vi "sub_pf_localization.vi"(11 "p-val out":T2) -> ()   [LabVIEW 2019]
uses:
  <vilib>/Analysis/Matrix/Datatypes/RealMatrix.ctl
  Ctrl/cmd_common.ctl
  <vilib>/Analysis/baseanly.llb/Real A x B.vi
  <vilib>/ptbypt/NI_PtbyPt.lvlib
  <vilib>/Analysis/NI_AALBase.lvlib
  <vilib>/Analysis/Matrix/NI_Matrix.lvlib
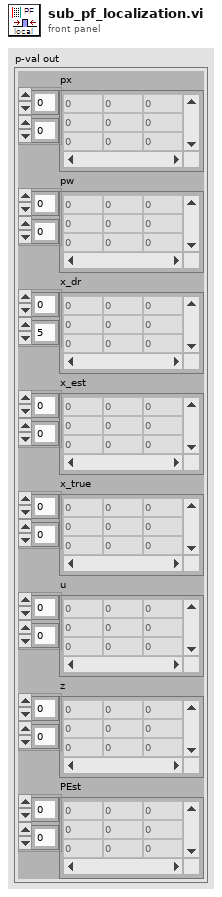
[diagram p1: front panel]
types:
  T1 = typedef "NI_Matrix.lvlib/RealMatrix.ctl" = dbl[][]
  T2 = cluster{"px":T1, "pw":T1, "x_dr":T1, "x_est":T1, "x_true":T1, "u":T1, "z":T1, "PEst":T1}
  T3 = typedef "cmd_common.ctl" = enum16{"read", "write"}
  T4 = cluster{"DT":dbl, "SIM_TIME":dbl, "MAX_RANGE":dbl, "NP":u32, "NTh":u32, "Q":T1, "R":T1, "Q_sim":T1, "R_sim":T1, "rf_id":cluster{"x":dbl, "y":dbl}[]}
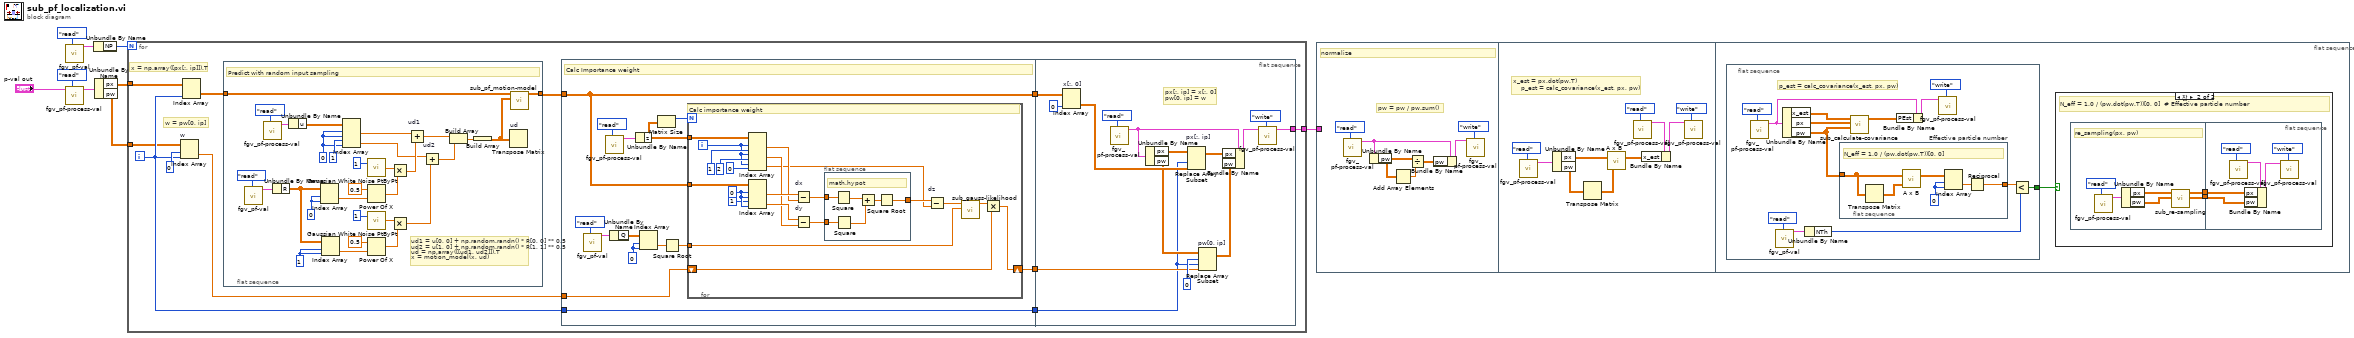
[diagram p0: block diagram]
diagram:
  n1 = call "fgv_pf-val.vi"("cmd"=cmd_common."read") -> ("pf-val out"=w7:T4)  [unwired: 10 in]
  n2 = call "fgv_pf-process-val.vi"("cmd"=cmd_common."read", "p-val"="p-val out") -> ("p-val out"=w2:T2)  [unwired: 9 in]
  n3 = Unbundle By Name(w7) -> ("NP"=w5:u32)
  n4 = Unbundle By Name(w2) -> ("px"=w4:T1, "pw"=w3:T1)
  n5 = for {
    N: w5 -> [_]
    tunnel: [w14] -> w8
    tunnel: w4 -> [w12]
    tunnel: w3 -> [w11]
    i -> [w13]
    # "x = np.array([px[:, ip]]).T"
    # "w = pw[0, ip]"
    n6 = Index Array "w"(array=w11, index (row)=0 ("인덱스 (행)"), index (col)=w13) -> (element=w18:dbl)
    n7 = Index Array(array=w12, index (col)=w13) -> (element=w10:T1)  [unwired: 1 in]
    n8 = flat-sequence {
      tunnel: [w23] -> w19
      tunnel: w10 -> [w22]
      frame #0 {
        w31 = 1 ("인덱스 (행)")
        w42 = 0 ("인덱스 (행)")
        w46 = 0 ("인덱스 (행)")
        # "ud1 = u[0, 0] + np.random.randn() * R[0, 0] ** 0.5\nud2 = u[1, 0] + np.random.randn() * R[1, 1] ** 0.5\nud = np.array([[ud1, ud2]]).T\nx = motion_model(x, ud)"
        # "Predict with random input sampling"
        n9 = call "fgv_pf-val.vi"("cmd"=cmd_common."read") -> ("pf-val out"=w43:T4)  [unwired: 10 in]
        n10 = call "fgv_pf-process-val.vi"("cmd"=cmd_common."read") -> ("p-val out"=w49:T2)  [unwired: 10 in]
        n11 = Unbundle By Name(w43) -> ("R"=w24:T1)
        n12 = Unbundle By Name(w49) -> ("u"=w48:T1)
        n13 = Index Array(array=w24, index (row)=w42, index (col)=w42) -> (element=w41:dbl)
        n14 = Index Array(array=w24, index (row)=w31, index (col)=w31) -> (element=w32:dbl)
        n15 = Index Array(array=w48, index (row) #1=w46, index (col) #1=w46, index (row) #2=1 ("인덱스 (행)"), index (col) #2=w46) -> (element #1=w36:dbl, element #2=w29:dbl)
        n16 = call <vilib>:"Gaussian White Noise PtByPt.vi"("standard deviation"=1 ("samples")) -> ("Gaussian white noise"=w38:dbl)  [unwired: 2 in]
        n17 = Power Of X(1:w41, 2:0.5 ("y")) -> (0:w39:dbl)
        n18 = call <vilib>:"Gaussian White Noise PtByPt.vi"("standard deviation"=1 ("samples")) -> ("Gaussian white noise"=w35:dbl)  [unwired: 2 in]
        n19 = Power Of X(1:w32, 2:0.5 ("y")) -> (0:w34:dbl)
        n20 = Multiply(x=w38, y=w39) -> (x*y=w37:dbl)
        n21 = Multiply(x=w35, y=w34) -> (x*y=w28:dbl)
        n22 = Add "ud1"(x=w36, y=w37) -> (x+y=w25:dbl)
        n23 = Add "ud2"(x=w29, y=w28) -> (x+y=w26:dbl)
        n24 = Build Array(w25, w26) -> (w27:dbl[])
        n25 = Build Array(w27) -> (w21:T1)
        n26 = Transpose Matrix "ud"(1:w21) -> ()  [unwired: 1 out]
        n27 = call "sub_pf_motion-model.vi"("u"=w21, "x_true"=w22) -> ("x_true out"=w23:T1)  [unwired: 9 in]
      }
    }
    n28 = flat-sequence {
      tunnel: w19 -> [w52]
      tunnel: w18 -> [w54]
      tunnel: w13 -> [w53]
      tunnel: [w53] -> w17
      tunnel: [w52] -> w16
      tunnel: [w51] -> w15
      tunnel: w15 -> [w96]
      tunnel: w16 -> [w102]
      tunnel: w17 -> [w95]
      tunnel: [w94] -> w14
      frame #0 {
        w57 = 0 ("인덱스 (행)")
        # "Calc Importance weight"
        n29 = call "fgv_pf-val.vi"("cmd"=cmd_common."read") -> ("pf-val out"=w59:T4)  [unwired: 10 in]
        n30 = call "fgv_pf-process-val.vi"("cmd"=cmd_common."read") -> ("p-val out"=w63:T2)  [unwired: 10 in]
        n31 = Unbundle By Name(w59) -> ("Q"=w58:T1)
        n32 = Unbundle By Name(w63) -> ("z"=w61:T1)
        n33 = Index Array(array=w58, index (row)=w57, index (col)=w57) -> (element=w56:dbl)
        n34 = Matrix Size(0:w61) -> (1:w62:i32)  [unwired: 1 out]
        n35 = Square Root(x=w56) -> (sqrt(x)=w55:dbl)
        n36 = for {
          N: w62 -> [_]
          tunnel: w52 -> [w85]
          tunnel: w61 -> [w82]
          tunnel: w55 -> [w69]
          shift-right: [w65] -> w51
          shift-left: w54 -> [w66]
          i -> [w68]
          w84 = 0 ("인덱스 (행)")
          # "Calc importance weight"
          n37 = Index Array(array=w82, index (row) #1=w68, index (col) #1=1 ("인덱스 (열)"), index (row) #2=w68, index (col) #2=2 ("인덱스 (열)"), index (row) #3=w68, index (col) #3=0 ("인덱스 (열)")) -> (element #1=w78:dbl, element #2=w76:dbl, element #3=w71:dbl)
          n38 = Index Array(array=w85, index (row) #1=w84, index (col) #1=w84, index (row) #2=1 ("인덱스 (행)"), index (col) #2=w84) -> (element #1=w79:dbl, element #2=w77:dbl)
          n39 = Subtract "dx"(x=w79, y=w78) -> (x-y=w74:dbl)
          n40 = Subtract "dy"(x=w77, y=w76) -> (x-y=w75:dbl)
          n41 = flat-sequence {
            tunnel: w75 -> [w91]
            tunnel: w74 -> [w90]
            tunnel: [w86] -> w72
            frame #0 {
              # "math.hypot"
              n42 = Square(x=w90) -> (x^2=w88:dbl)
              n43 = Square(x=w91) -> (x^2=w87:dbl)
              n44 = Add(x=w88, y=w87) -> (x+y=w89:dbl)
              n45 = Square Root(x=w89) -> (sqrt(x)=w86:dbl)
            }
          }
          n46 = Subtract "dz"(x=w72, y=w71) -> (x-y=w70:dbl)
          n47 = call "sub_gauss-likelihood.vi"("sigma"=w69, "x"=w70) -> ("p"=w67:dbl)  [unwired: 9 in]
          n48 = Multiply ("Multiply.vi")(x=w67, y=w66) -> (x*y=w65:dbl)
        }
      }
      frame #1 {
        # "px[:, ip] = x[:, 0]\npw[0, ip] = w"
        n49 = Index Array "x[:, 0]"(array=w102, index (col)=0) -> (element=w99:T1)  [unwired: 1 in]
        n50 = call "fgv_pf-process-val.vi"("cmd"=cmd_common."read") -> ("p-val out"=w103:T2)  [unwired: 10 in]
        n51 = Unbundle By Name(w103) -> ("px"=w100:T1, "pw"=w98:T1)
        n52 = Replace Array Subset "px[:, ip]"(array=w100, new element=w99, index (col)=w95) -> (w92:T1)  [unwired: 1 in]
        n53 = Replace Array Subset "pw[0, ip]"(array=w98, new element=w96, index (row)=0 ("index (col)"), index (col)=w95) -> (w93:T1)
        n54 = Bundle By Name(cluster=w103, "px"=w92, "pw"=w93) -> (w106:T2)
        n55 = call "fgv_pf-process-val.vi"("cmd"=cmd_common."write", "p-val"=w106) -> ("p-val out"=w94:T2)  [unwired: 9 in]
      }
    }
  }
  n56 = flat-sequence {
    tunnel: w8 -> [_]
    frame #0 {
      # "pw = pw / pw.sum()"
      # "normalize"
      n57 = call "fgv_pf-process-val.vi"("cmd"=cmd_common."read") -> ("p-val out"=w112:T2)  [unwired: 10 in]
      n58 = Unbundle By Name(w112) -> ("pw"=w110:T1)
      n59 = Add Array Elements(numeric array=w110) -> (sum=w109:dbl)
      n60 = Divide(x=w110, y=w109) -> (x/y=w111:T1)
      n61 = Bundle By Name(cluster=w112, "pw"=w111) -> (w113:T2)
      n62 = call "fgv_pf-process-val.vi"("cmd"=cmd_common."write", "p-val"=w113) -> ()  [unwired: 9 in, 1 out]
    }
    frame #1 {
      # "x_est = px.dot(pw.T)\n    p_est = calc_covariance(x_est, px, pw)"
      n63 = call "fgv_pf-process-val.vi"("cmd"=cmd_common."read") -> ("p-val out"=w123:T2)  [unwired: 10 in]
      n64 = Unbundle By Name(w123) -> ("px"=w122:T1, "pw"=w121:T1)
      n65 = Transpose Matrix(1:w121) -> (0:w120:T1)
      n66 = call-poly <vilib>:"A x B.vi"("B"=w120, "A"=w122) -> ("A x B"=w117:T1)  [unwired: 1 out]
      n67 = call "fgv_pf-process-val.vi"("cmd"=cmd_common."read") -> ("p-val out"=w118:T2)  [unwired: 10 in]
      n68 = Bundle By Name(cluster=w118, "x_est"=w117) -> (w119:T2)
      n69 = call "fgv_pf-process-val.vi"("cmd"=cmd_common."write", "p-val"=w119) -> ()  [unwired: 9 in, 1 out]
    }
    frame #2 {
      n70 = flat-sequence {
        tunnel: [w129] -> w124
        frame #0 {
          # "p_est = calc_covariance(x_est, px, pw)"
          n71 = call "fgv_pf-process-val.vi"("cmd"=cmd_common."read") -> ("p-val out"=w127:T2)  [unwired: 10 in]
          n72 = call "fgv_pf-val.vi"("cmd"=cmd_common."read") -> ("pf-val out"=w131:T4)  [unwired: 10 in]
          n73 = Unbundle By Name(w127) -> ("x_est"=w135:T1, "px"=w136:T1, "pw"=w134:T1)
          n74 = Unbundle By Name(w131) -> ("NTh"=w130:u32)
          n75 = flat-sequence "Effective particle number" {
            tunnel: w134 -> [w143]
            tunnel: [w138] -> w132
            frame #0 {
              w140 = 0 ("index (row)")
              # "N_eff = 1.0 / (pw.dot(pw.T))[0, 0]"
              n76 = Transpose Matrix(1:w143) -> (0:w142:T1)
              n77 = call-poly <vilib>:"A x B.vi"("B"=w142, "A"=w143) -> ("A x B"=w141:T1)  [unwired: 1 out]
              n78 = Index Array(array=w141, index (row)=w140, index (col)=w140) -> (element=w139:dbl)
              n79 = Reciprocal(x=w139) -> (1/x=w138:dbl)
            }
          }
          n80 = call "sub_calculate-covariance.vi"("pw"=w134, "px"=w136, "x_est"=w135) -> ("cov out"=w126:T1)  [unwired: 8 in]
          n81 = Bundle By Name(cluster=w127, "PEst"=w126) -> (w125:T2)
          n82 = call "fgv_pf-process-val.vi"("cmd"=cmd_common."write", "p-val"=w125) -> ()  [unwired: 9 in, 1 out]
          n83 = Less?(x=w132, y=w130) -> (x < y?=w129:bool)
        }
      }
      n84 = case shown="참" w124 {
        frame False {
        }
        frame True {
          # "N_eff = 1.0 / (pw.dot(pw.T))[0, 0]  # Effective particle number"
          n85 = flat-sequence {
            tunnel: [w147] -> w145
            tunnel: [w146] -> w144
            tunnel: w145 -> [w155]
            tunnel: w144 -> [w154]
            frame #0 {
              # "re_sampling(px, pw)"
              n86 = call "fgv_pf-process-val.vi"("cmd"=cmd_common."read") -> ("p-val out"=w151:T2)  [unwired: 10 in]
              n87 = Unbundle By Name(w151) -> ("px"=w148:T1, "pw"=w149:T1)
              n88 = call "sub_re-sampling.vi"("pw"=w149, "px"=w148) -> ("pw"=w146:T1, "px out"=w147:T1)  [unwired: 8 in]
            }
            frame #1 {
              n89 = call "fgv_pf-process-val.vi"("cmd"=cmd_common."read") -> ("p-val out"=w157:T2)  [unwired: 10 in]
              n90 = Bundle By Name(cluster=w157, "px"=w155, "pw"=w154) -> (w156:T2)
              n91 = call "fgv_pf-process-val.vi"("cmd"=cmd_common."write", "p-val"=w156) -> ()  [unwired: 9 in, 1 out]
            }
          }
        }
      }
    }
  }
